vi "Noise.vi"(10 "AWGN (dB)":dbl, 11 "Dynamic Data":dynamicdata(waveform)) -> (3 "DC with Gaussian Noise":dynamicdata(waveform))   [LabVIEW 2013]
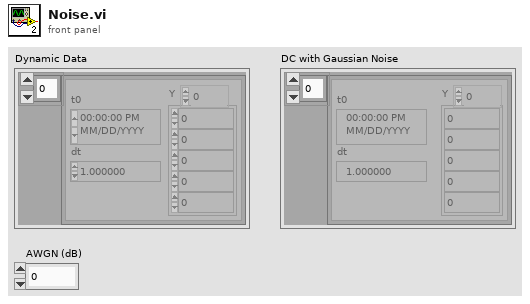
[diagram p1: front panel]
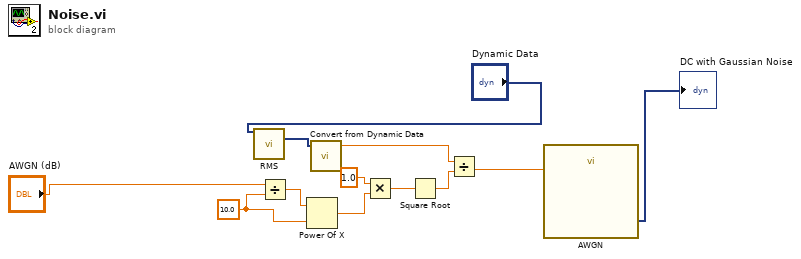
[diagram p0: block diagram]
diagram:
  w8 = 10.0
  n1 = call "RMS"("Signals"="Dynamic Data") -> ("RMS"=w12:dynamicdata)  [unwired: 13 in, 1 out]
  n2 = Divide(x="AWGN (dB)", y=w8) -> (x/y=w2:dbl)
  n3 = Power Of X(1:w8, 2:w2) -> (0:w4:dbl)
  n4 = call "Convert from Dynamic Data"("Dynamic Data Type"=w12) -> ("Scalar"=w7:dbl)  [unwired: 3 in]
  n5 = Multiply(x=1.0, y=w4) -> (x*y=w5:dbl)
  n6 = Square Root(x=w5) -> (sqrt(x)=w6:dbl)
  n7 = Divide(x=w7, y=w6) -> (x/y=w11:dbl)
  n8 = call "AWGN"("Standard deviation"=w11) -> ("DC with Gaussian Noise"=→"DC with Gaussian Noise":dynamicdata)  [unwired: 13 in, 1 out]
